vi "FP Color Strategy.vi"() -> ()   [LabVIEW 2021]
uses:
  Color Strategy/Color Strategy.lvclass
panel:
  in  "Color Strategy.lvclass":refnum<class "Color Strategy.lvclass">
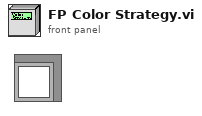
[diagram p1: front panel]
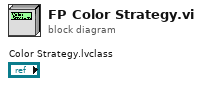
[diagram p0: block diagram]
diagram:
